vi "Clear screens (SubVI).vi"(11 "String refs":refnum<vi>[](array[refnum])) -> (3 "String refs out":refnum<vi>[](array[refnum]))   [LabVIEW 2021]
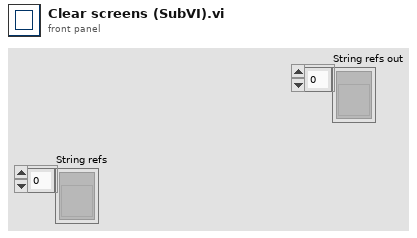
[diagram p1: front panel]
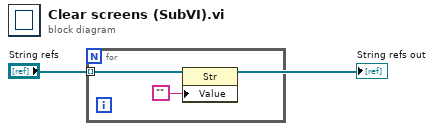
[diagram p0: block diagram]
diagram:
  n1 = for {
    tunnel: "String refs" -> [w3] mode=indexing
    n2 = property class="Str"(reference=w3, "Value"="") -> ()  [unwired: 1 in, 2 out]
  }
  "String refs out" <- "String refs"
